vi "Result View.vi"() -> ()   [LabVIEW 2020, in "Test Result View.lvclass"]
uses:
  Test Result View/Test Result View.lvclass
  Test Result View/Test Result View.lvclass/Test Result View.ctl
panel:
  in  "Test Results":string[](tree)
  in  "Filter fails":bool
  out "Description":string
  out "error out":errorcluster
  in  "error in (no error)":errorcluster
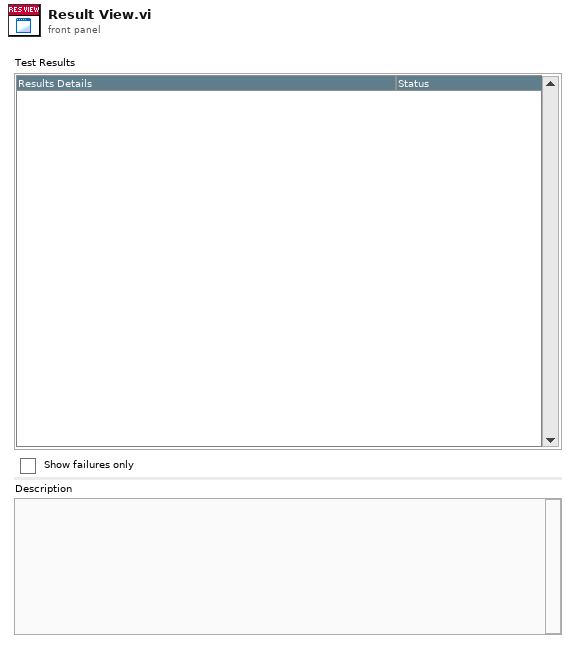
[diagram p1: front panel]
types:
  T1 = cluster{"Message":string, "Message Data":variant}
  T2 = enum32{"Invalid", "Standard", "Closed", "Hidden", "Minimized", "Maximized"}
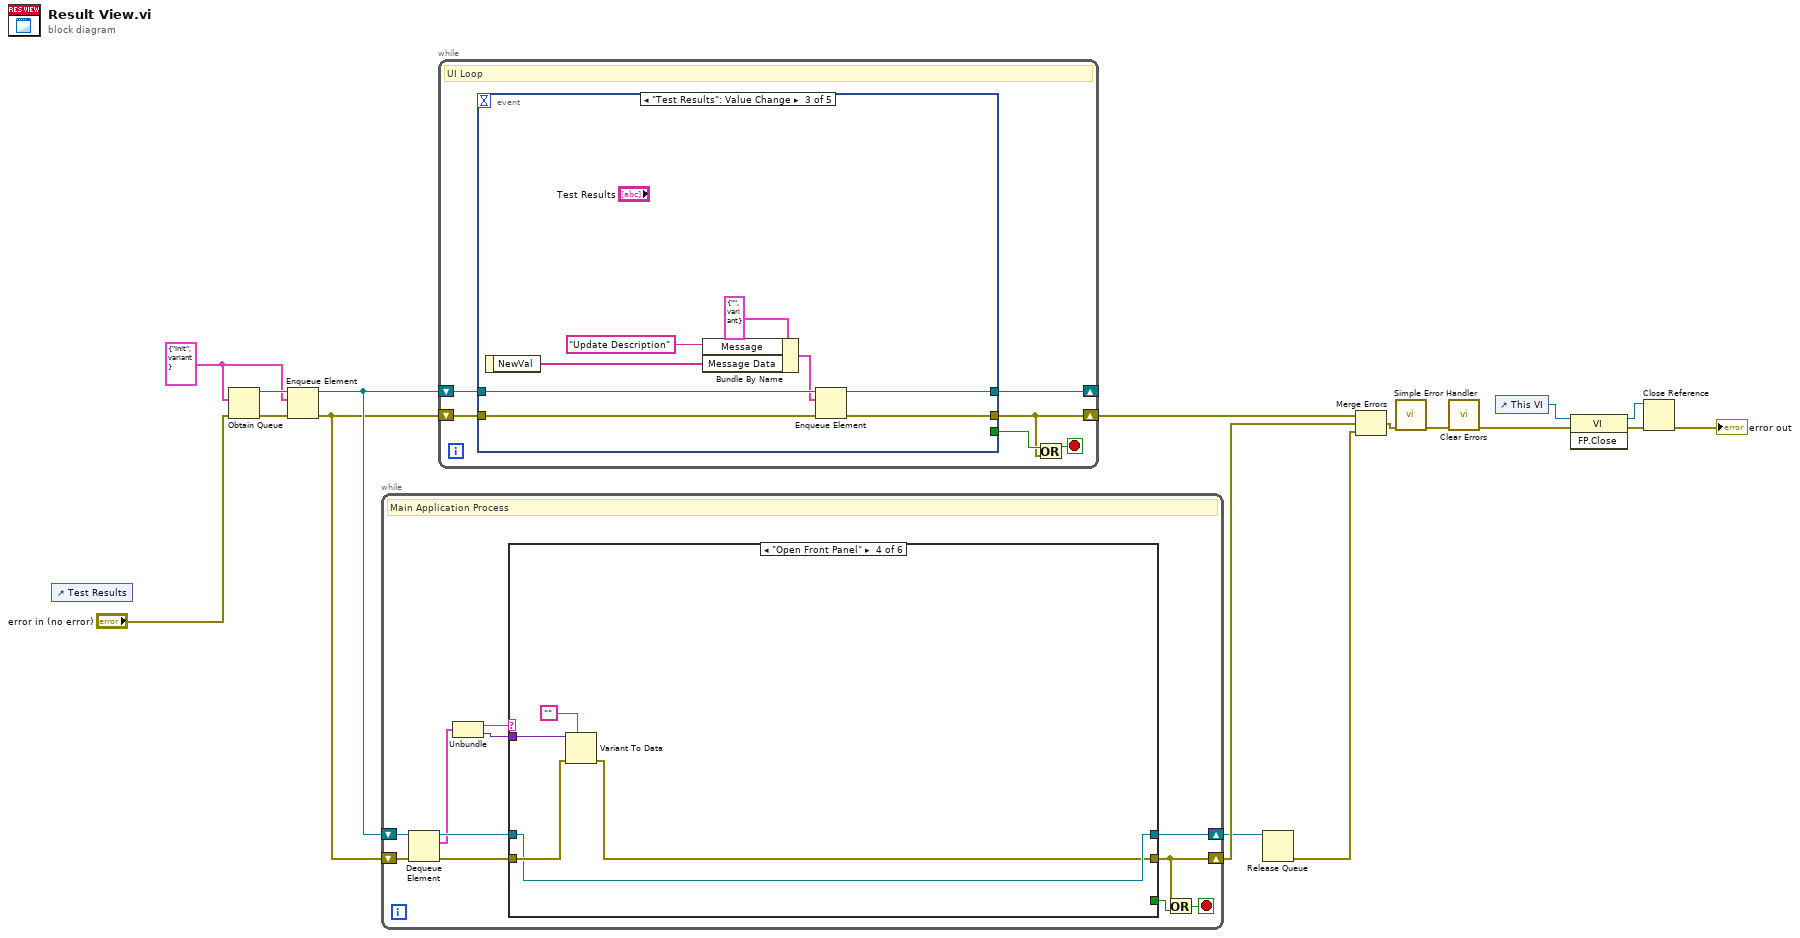
[diagram p0: block diagram]
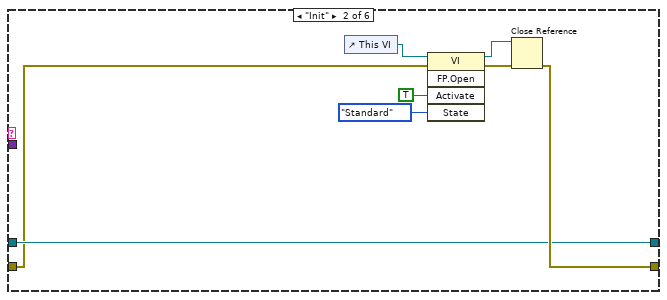
[diagram p3: hidden frame]
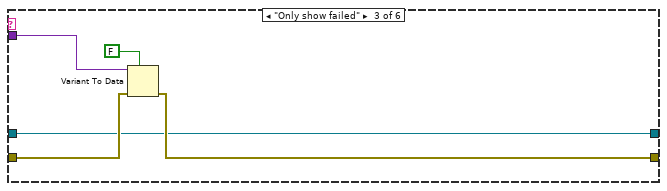
[diagram p4: hidden frame]
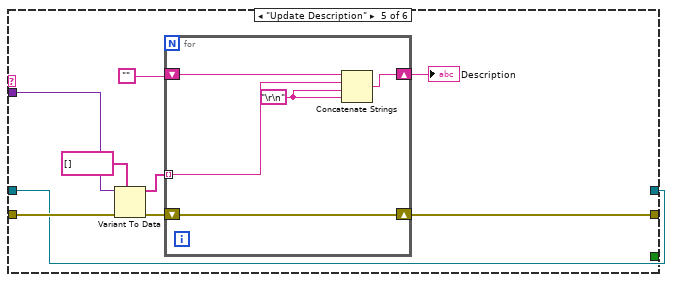
[diagram p5: hidden frame]
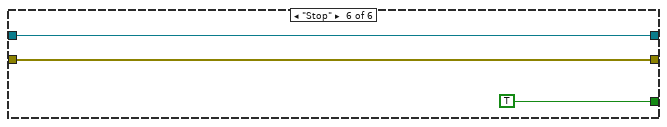
[diagram p6: hidden frame]
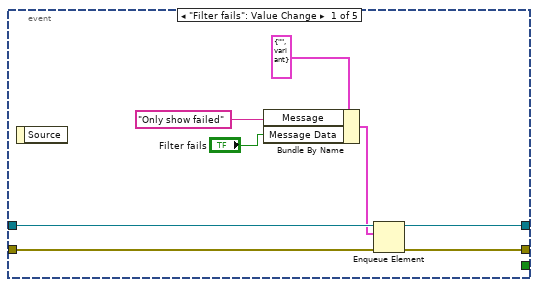
[diagram p7: hidden frame]
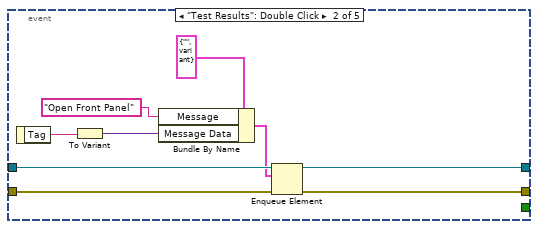
[diagram p8: hidden frame]
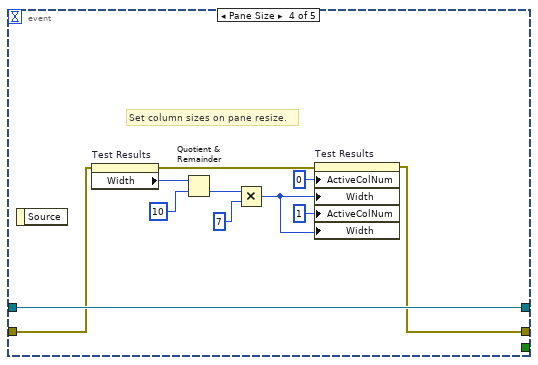
[diagram p9: hidden frame]
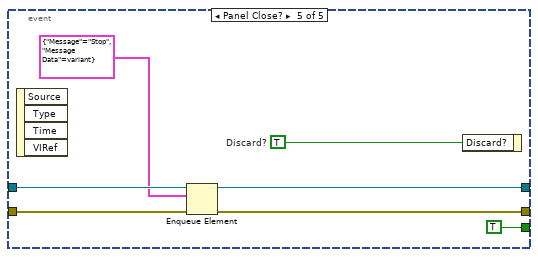
[diagram p10: hidden frame]
diagram:
  w1 = T1 {"Message"="Init", "Message Data"=variant} ("element")
  n1 = control-ref of="Test Results"() -> ()  [unwired: 1 out]
  n2 = Obtain Queue(element data type=w1, error in (no error)="error in (no error)") -> (queue out=w13:refnum<queue>, error out=w11:errorcluster)  [unwired: 3 in, 1 out]
  n3 = Enqueue Element(queue=w13, element=w1, error in (no error)=w11) -> (queue out=w12:refnum<queue>, error out=w10:errorcluster)  [unwired: 1 in, 1 out]
  n4 = while {
    shift-right: [w18] -> w17
    shift-left: w10 -> [w27]
    shift-right: [w23] -> w6
    shift-left: w12 -> [w28]
    stop <- w19 stop-if-true
    # "Main Application Process"
    n5 = Dequeue Element(queue=w28, error in (no error)=w27) -> (queue out=w26:refnum<queue>, element=w22:T1, error out=w25:errorcluster)  [unwired: 1 in, 1 out]
    n6 = Unbundle(w22) -> ("Message"=w21:string, "Message Data"=w20:variant)
    n7 = case shown="\"Open Front Panel\"" w21 {
      tunnel: w26 -> [w29 w32 w39 w45 w49 w63]
      tunnel: [w29 w32 w39 w45 w49 w63] -> w23
      tunnel: w25 -> [w30 w31 w43 w48 w57 w64]
      tunnel: [w30 w33 w40 w44 w52 w64] -> w18
      tunnel: [_ _ _ _ _ TRUE] -> w24
      tunnel: w20 -> [_ _ w42 w47 w56 _]
      frame Default {
      }
      frame "Init" {
        n8 = control-ref of="This VI"() -> (w36:refnum<vi>)
        n9 = invoke on="Invoke Node" class="VI" method="FP.Open"(reference=w36, error in=w31, "Activate"=TRUE ("Activate?"), "State"=T2."Standard") -> (reference out=w34:refnum<vi>, error out=w35:errorcluster)  [unwired: 1 in, 3 out]
        n10 = Close Reference(reference=w34, error in (no error)=w35) -> (error out=w33:errorcluster)
      }
      frame "Only show failed" {
        n11 = Variant To Data(error in=w43, type=FALSE, Variant=w42) -> (error out=w40:errorcluster)  [unwired: 1 out]
      }
      frame "Open Front Panel" {
        n12 = Variant To Data(error in=w48, type="" ("Empty String Constant"), Variant=w47) -> (error out=w44:errorcluster)  [unwired: 1 out]
      }
      frame "Update Description" {
        n13 = Variant To Data(error in=w57, type=string[] [], Variant=w56) -> (data=w54:string[], error out=w53:errorcluster)
        n14 = for {
          tunnel: w54 -> [w62] mode=indexing
          shift-right: [w61] -> w52
          shift-left: w53 -> [w61]
          shift-right: [w60] -> w50
          shift-left: "" ("Empty String Constant") -> [w59]
          w58 = "\r\n" ("End of Line Constant")
          n15 = Concatenate Strings(w59, w62, w58, w58) -> (w60:string)
        }
        "Description" <- w50
      }
      frame "Stop" {
      }
    }
    n16 = Or(x=w18, y=w24) -> (x .or. y?=w19:bool)
  }
  n17 = while {
    shift-right: [w66] -> w16
    shift-left: w10 -> [w70]
    shift-right: [w68] -> _
    shift-left: w12 -> [w71]
    stop <- w67 stop-if-true
    # "UI Loop"
    n18 = event shown="[2] \"Test Results\": Value Change" {
      selector: _ -> [_ _ _ _ _]
      dyn-events: _ -> [_ _ _ _ _]
      timeout: _ -> [_ _ _ _ _]
      tunnel: w71 -> [w79 w88 w96 w107 w113]
      tunnel: w70 -> [w77 w87 w95 w97 w110]
      tunnel: [w76 w85 w94 w98 w111] -> w66
      tunnel: [w78 w86 w93 w107 w112] -> w68
      tunnel: [_ _ _ _ TRUE] -> w69
      event "Filter fails": Value Change {
        n19 = event-data() -> ()  [unwired: 1 in, 1 out]
        n20 = Bundle By Name(cluster=T1 {"Message"="", "Message Data"=variant} ("element"), "Message"="Only show failed", "Message Data"="Filter fails") -> (w74:T1)
        n21 = Enqueue Element(queue=w79, element=w74, error in (no error)=w77) -> (queue out=w78:refnum<queue>, error out=w76:errorcluster)  [unwired: 1 in, 1 out]
      }
      event "Test Results": Double Click {
        n22 = event-data() -> ("Tag"=w84:string)  [unwired: 1 in]
        n23 = To Variant(anything=w84) -> (Variant=w81:variant)
        n24 = Bundle By Name(cluster=T1 {"Message"="", "Message Data"=variant} ("element"), "Message"="Open Front Panel", "Message Data"=w81) -> (w82:T1)
        n25 = Enqueue Element(queue=w88, element=w82, error in (no error)=w87) -> (queue out=w86:refnum<queue>, error out=w85:errorcluster)  [unwired: 1 in, 1 out]
      }
      event "Test Results": Value Change {
        n26 = event-data() -> ("NewVal"=w89:string[])  [unwired: 1 in]
        n27 = Bundle By Name(cluster=T1 {"Message"="", "Message Data"=variant} ("element"), "Message"="Update Description", "Message Data"=w89) -> (w91:T1)
        n28 = Enqueue Element(queue=w96, element=w91, error in (no error)=w95) -> (queue out=w93:refnum<queue>, error out=w94:errorcluster)  [unwired: 1 in, 1 out]
      }
      event Pane Size {
        # "Set column sizes on pane resize."
        n29 = event-data() -> ()  [unwired: 1 in, 1 out]
        n30 = property on="Test Results" class="Tree (strict)"(error in=w97) -> (error out=w99:errorcluster, "Width"=w100:u32)  [unwired: 1 in, 1 out]
        n31 = Quotient & Remainder(x=w100, y=u32 10) -> (floor(x/y)=w104:u32)  [unwired: 1 out]
        n32 = Multiply(x=w104, y=u32 7) -> (x*y=w101:u32)
        n33 = property on="Test Results" class="Tree (strict)"(error in=w99, "ActiveColNum"=0 ("Active Cell:Active Column Number"), "Width"=w101, "ActiveColNum"=1 ("Active Cell:Active Column Number"), "Width"=w101) -> (error out=w98:errorcluster)  [unwired: 1 in, 1 out]
      }
      event Panel Close? {
        w114 = TRUE  # Discard?
        n34 = event-data() -> ()  [unwired: 1 in, 4 out]
        n35 = Enqueue Element(queue=w113, element=T1 {"Message"="Stop", "Message Data"=variant}, error in (no error)=w110) -> (queue out=w112:refnum<queue>, error out=w111:errorcluster)  [unwired: 1 in, 1 out]
        n36 = event-data ("Event Filter Node")("Discard?"=w114) -> ()  [unwired: 1 in, 1 out]
      }
    }
    n37 = Or(x=w69, y=w66) -> (x .or. y?=w67:bool)
  }
  n38 = Release Queue(queue=w6) -> (error out=w5:errorcluster)  [unwired: 2 in, 2 out]
  n39 = Merge Errors(w16, w17, w5) -> (w15:errorcluster)
  n40 = call <vilib>:"Simple Error Handler.vi"("error in (no error)"=w15) -> ("error out"=w4:errorcluster)  [unwired: 4 in, 4 out]
  n41 = call <vilib>:"Clear Errors.vi"("error in (no error)"=w4) -> ("error out"=w3:errorcluster)  [unwired: 5 in, 1 out]
  n42 = control-ref of="This VI"() -> (w7:refnum<vi>)
  n43 = invoke on="Invoke Node" class="VI" method="FP.Close"(reference=w7, error in=w3) -> (reference out=w9:refnum<vi>, error out=w8:errorcluster)  [unwired: 1 in, 1 out]
  n44 = Close Reference(reference=w9, error in (no error)=w8) -> (error out=→"error out":errorcluster)
